vi "SPARC4_GEI.vi"() -> ()   [LabVIEW 2018]
uses:
  SPARC4_GUI/SPARC4_GEI.lvclass
  SPARC4_GUI/SPARC4_GEI.lvclass/SPARC4_GEI.ctl
  Interface/Interface.lvclass/Interface.ctl
  Channel GUI/Channel GEI.lvclass/Channel GEI.ctl
  State Machine/State Machine.lvclass/State Machine.ctl
  Channel GUI/Channel GEI.lvclass
  State Machine/State Machine.lvclass
  RxTx/RxTx.lvclass
  Interface/Interface.lvclass
panel:
  out "Error Message":string
  in  "Tab Control 2":enum32{"Front Panel", "Setup Panel"}(tab)
  in  "Number of channels":u16=1 min=1
  in  "FOCUS":bool caption="TEST"
  in  "TEST":bool
  in  "ZERO":bool caption="BIAS"
  in  "FLAT":bool
  in  "OBJECT":bool caption="SCIENCE"
  in  "DARK":bool caption="TEST"
  in  "Suffix:":string
  in  "Comment:":string="Go SPARC4!"
  in  "Filter":u16(ring) items=["Clear", "U", "B", "V", "R", "I"]
  out "Exposições realizadas":u16(slide)=1 max=2 scale=0.0..1.0
  out "Exposing":bool
  in  "Dummy":bool
  out "Camera On/Off":bool
  in  "Abort Acquisition":bool
  in  "Stop Acquisition":bool
  in  "Cubes":u32=1 min=1
  in  "Frames":u16=1 min=1
  in  "Send Message":bool
  out "Response:":string
  in  "Command:":string
  out "Last image":string="CH1"
  out "CCD Status":string
  out "Exp Time":sgl
  out "Temperature":i16
  out "Serial Number":u16
  out "Temperature Status":string
  in  "Exposure Time":sgl=1.0 min=1e-05
  in  "Acquire":bool
  in  "Stop Application":bool
  in  "TCS Simulated/Real":bool
  in  "EM Mode":u8(ring)=1 items=["Electron Multiplying", "Conventional"]
  in  "EM Gain":u16=2
  in  "Temperature 2":i16=20 min=-80 max=20
  in  "Cooler ON/OFF":u16(ring) items=["Cooler OFF", "Cooler ON"]
  in  "Readout Rate":u8(ring) items=["1 MHz", "0.1 MHz"]
  in  "Exposure Time 2":sgl=1.0 min=1e-05
  in  "Pre-amp gain":u8(ring) items=["Gain 1", "Gain 2"]
  in  "Frames 2":u16=1 min=1
  in  "Frame Tansfer":bool=TRUE
  in  "Trigger Mode":u16(ring) items=["Internal", "External", "N/A", "N/A", "N/A", "N/A", "External Start", "External Exposure (Bulb)", "N/A", "External FVB EM", "Software", "N/A", "External Charge Shifting"]
  in  "Vertical Shift Speed":u16=3
  in  "Read Mode":u16(ring)=4 items=["Full Vertical Binning", "Multi-Track", "Random-Track", "Single-Track", "Image"]
  in  "Vertical Clock Voltagem":u16
  in  "AD Channel":u16
  in  "Acquisition Mode":u16(ring)=3 items=["Reserved", "Single Scan", "Accumulate", "Kinetic", "Fast Kinetic", "Run till abort", "Reserved", "Reserved", "Reserved", "Time Delayed Integration"]
  in  "Shutter TTL":u16(ring) items=["TTL Low", "TTL High"]
  in  "Shutter Time":u16=50
  in  "Shutter Mode":u8(ring)=2 items=["Fully Auto", "OPEN", "CLOSED"]
  in  "Sub Image":T1(radio)=enum."1024 x 1024"
  in  "Final Line":u16=1024
  in  "Final Column":u16=1024
  in  "Initial Cloumn":u16=1
  in  "Initial Line":u16=1
  in  "Binning":u16=1
  # "SPARC4  ACS\nGraphical Engineering Interface (GEI)"
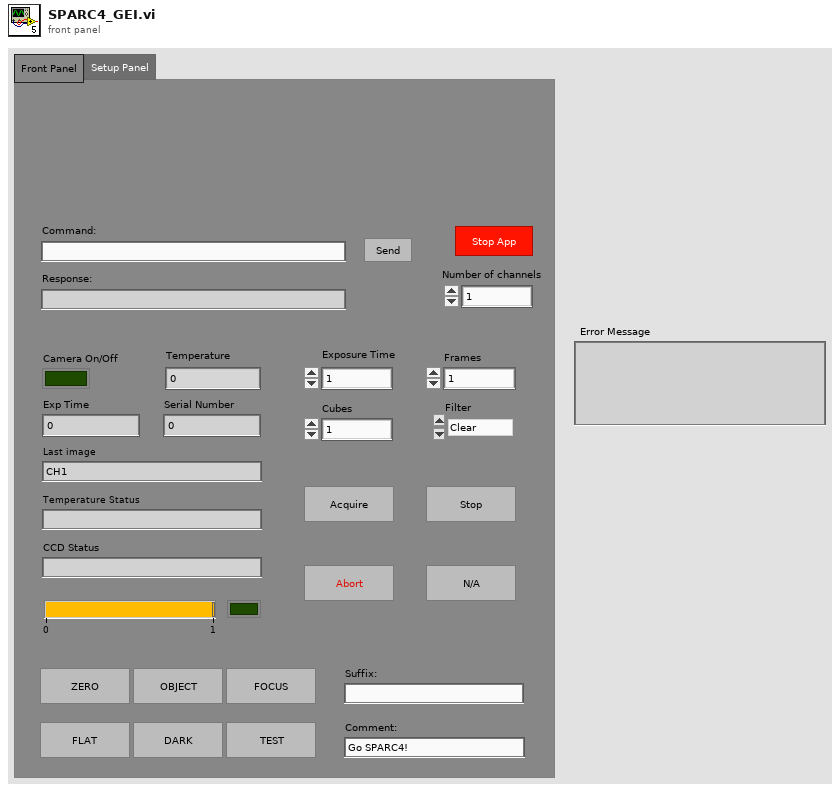
[diagram p1: front panel]
types:
  T1 = enum32{"256 x 256", "512 x 512", "1024 x 1024", "Custom"}
  T2 = enum8{"Enabled", "Disabled", "Disabled and Grayed Out"}
  T3 = cluster{"CUBE_EXPOSURE_TIME":sgl, "CUBES_DONE":u16, "LAST_IMAGE_NAME":string, "DISK_SPACE":u16, "FRAMES_DONE":u16, "CCD_STATUS":string, "CURRENT_TEMPERATURE":i16, "TEMPERATURE_STATUS":string, "FRAME_EXPOSURE_TIME":dbl, "CCD_POWER_STATUS":bool, "SERIAL_NUMBER":u16, "ACQUIRING":bool}
  T4 = cluster{"PREAMP":u16, "READOUT_RATE":u16, "EM_GAIN":u16, "VBIN":u16, "INITIAL_LINE":u16, "INITIAL_COLUMN":u16, "FINAL_LINE":u16, "FINAL_COLUMN":u16, "TRIGGER_MODE":u16, "HBIN":u16, "SHUTTER_TTL":u16, "SHUTTER_MODE":u16, "SHUTTER_OPENING_TIME":u16, "SHUTTER_CLOSING_TIME":u16, "VERTICAL_SHIFT_SPEED":u16, "READ_MODE":u16, "FRAME_TRANSFER":bool, "VERTICAL_CLOCK_VOLTAGE":u16, "ACQUISITION_MODE":u16, "AD_CHANNEL":u16, "EM_MODE":u16}
  T5 = cluster{"COOLER_POWER_STATUS":u16, "TEMP":i32, "EXPTIME":dbl, "#FRAMES":u32, "#CUBES":u32}
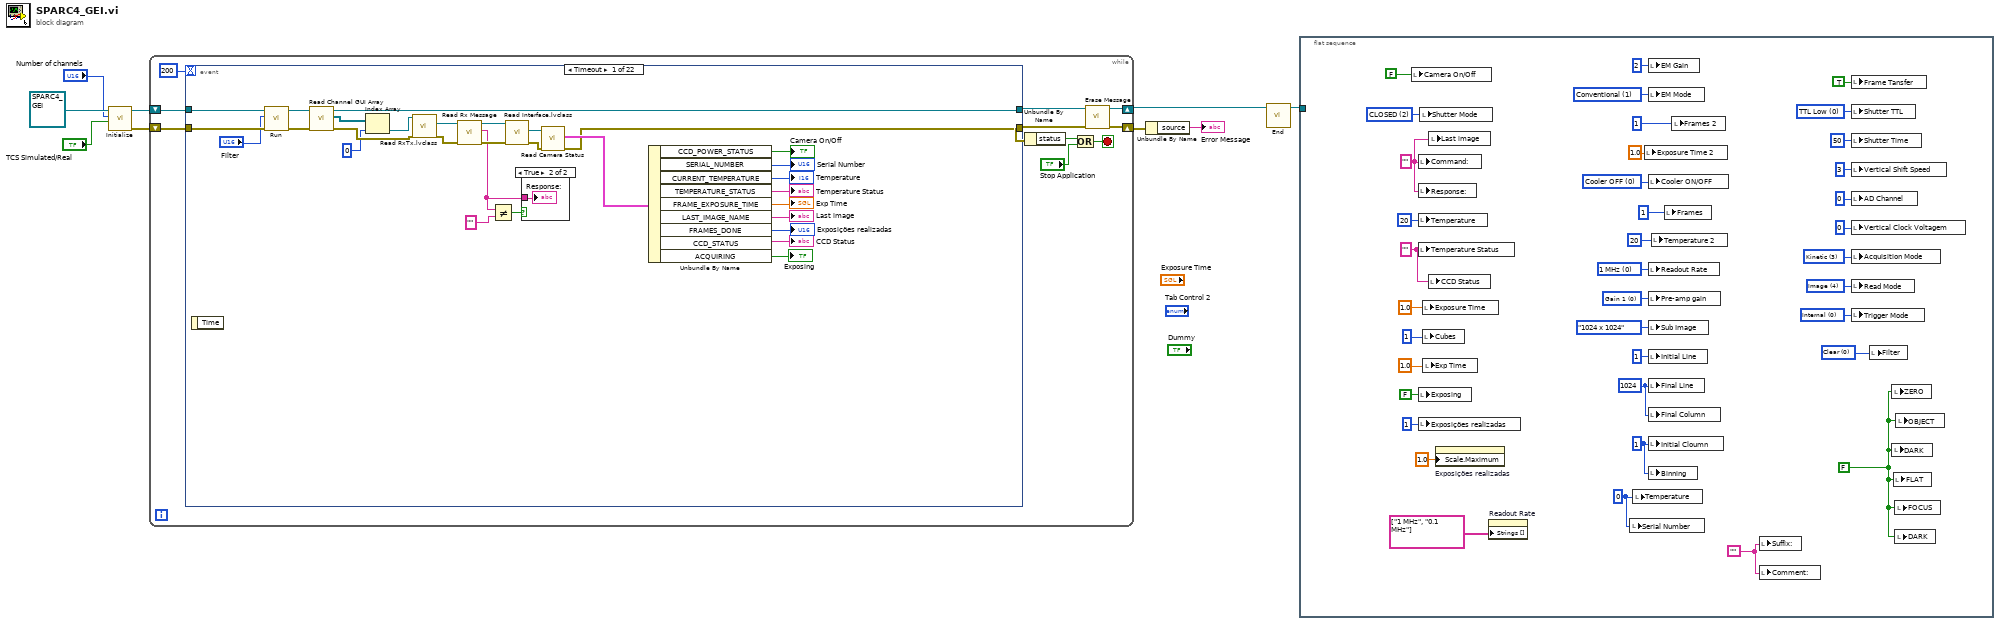
[diagram p0: block diagram]
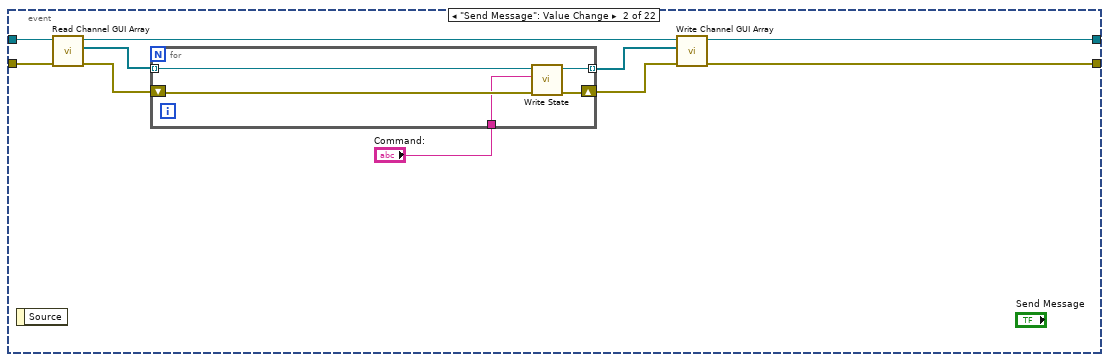
[diagram p3: hidden frame]
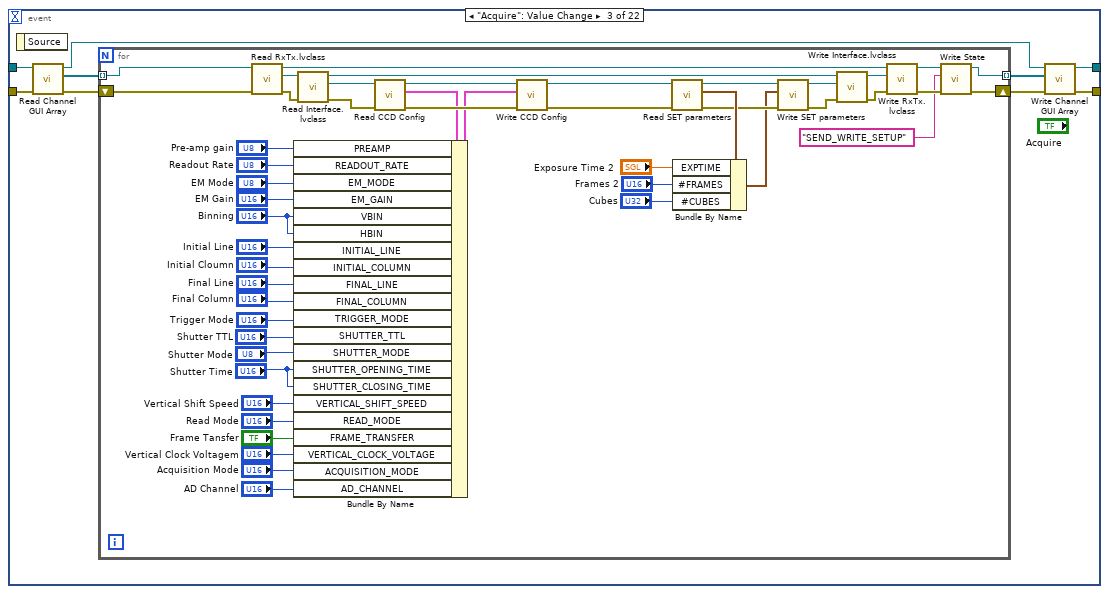
[diagram p4: hidden frame]
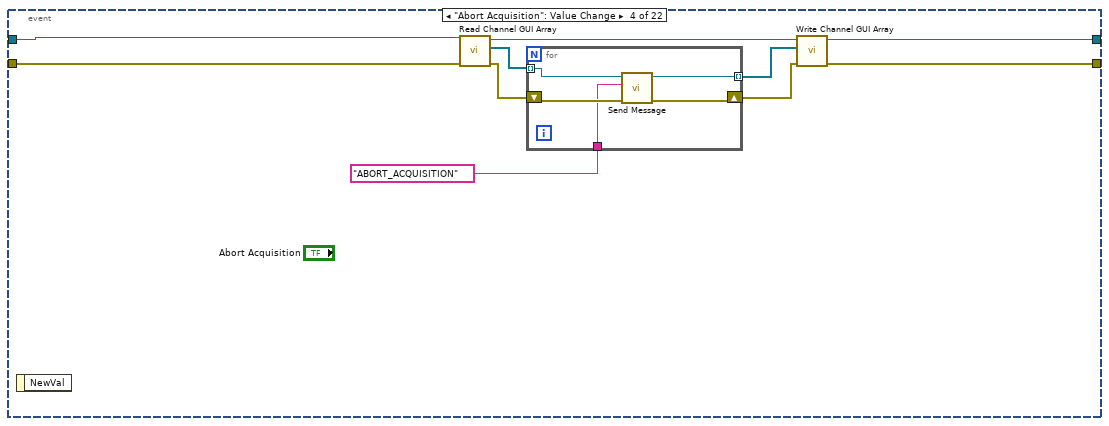
[diagram p5: hidden frame]
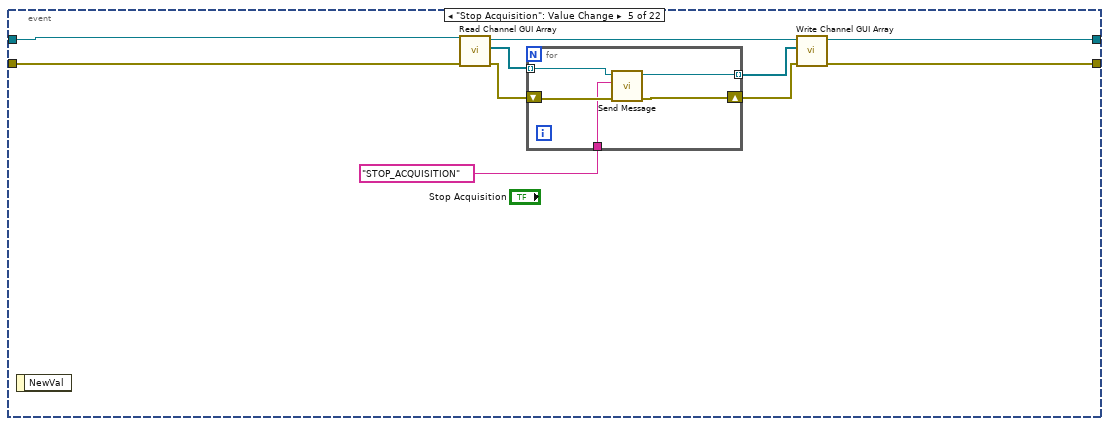
[diagram p6: hidden frame]
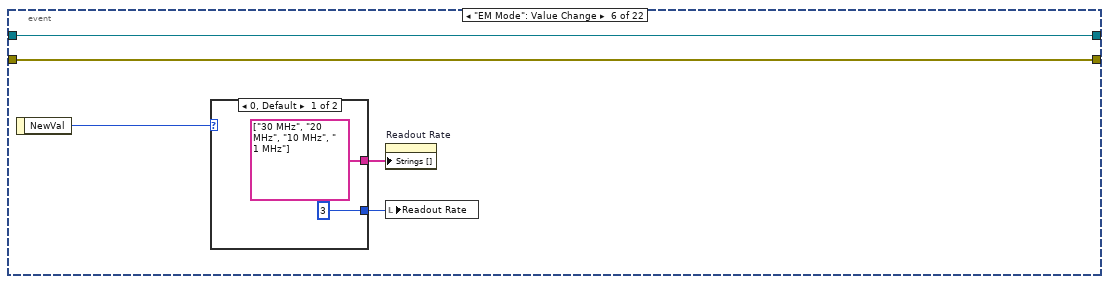
[diagram p7: hidden frame]
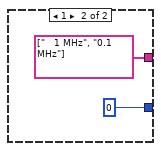
[diagram p8: hidden frame]
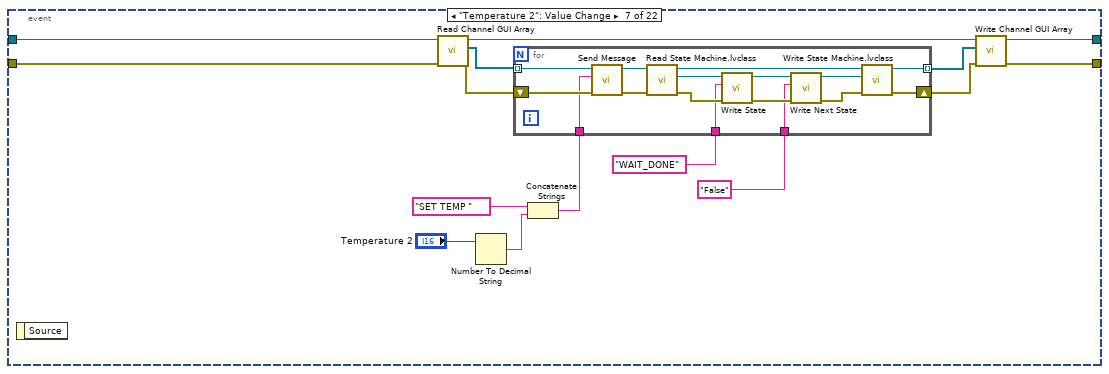
[diagram p9: hidden frame]
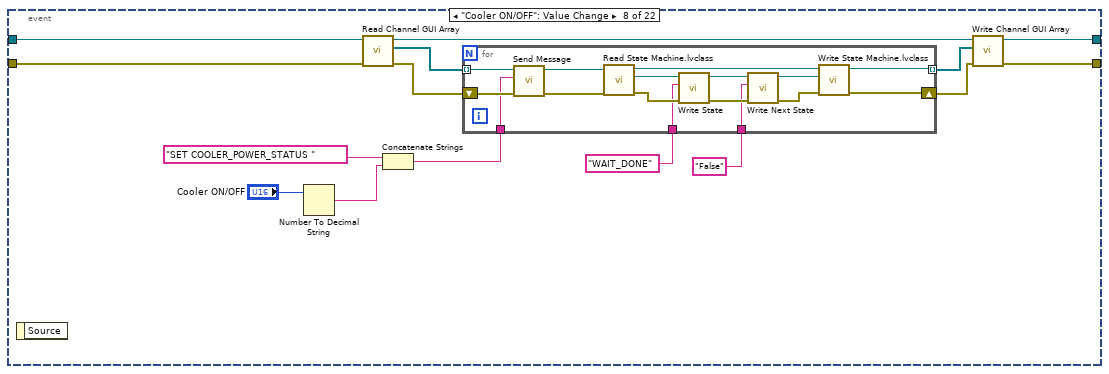
[diagram p10: hidden frame]
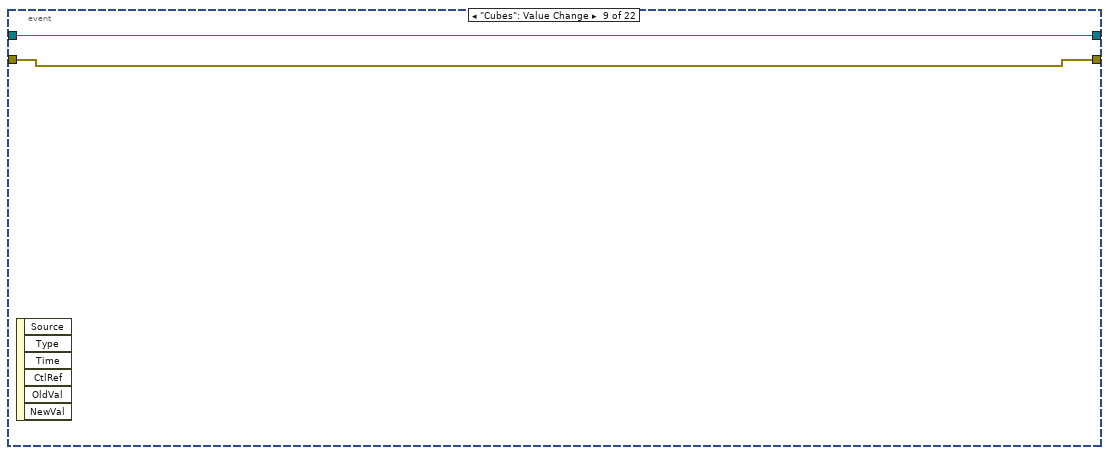
[diagram p11: hidden frame]
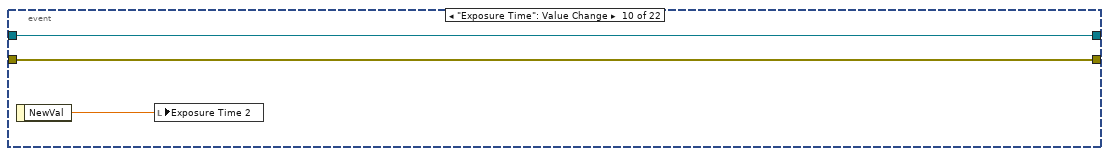
[diagram p12: hidden frame]
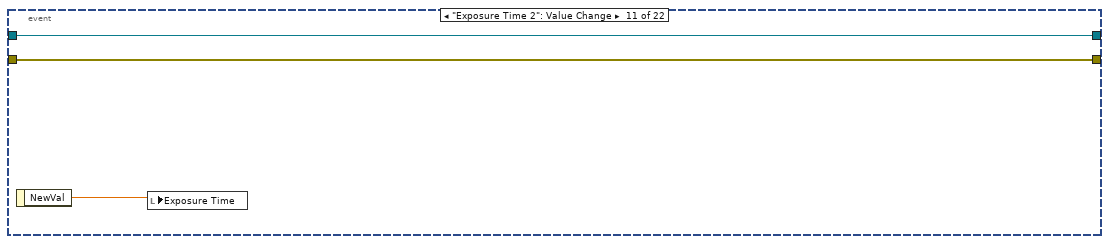
[diagram p13: hidden frame]
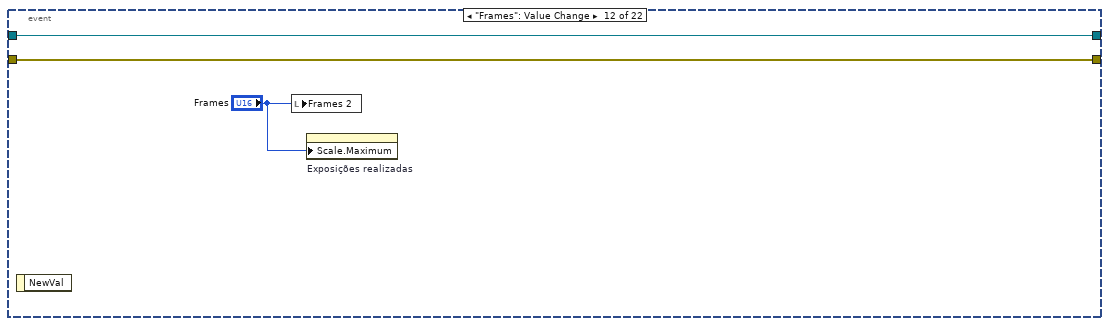
[diagram p14: hidden frame]
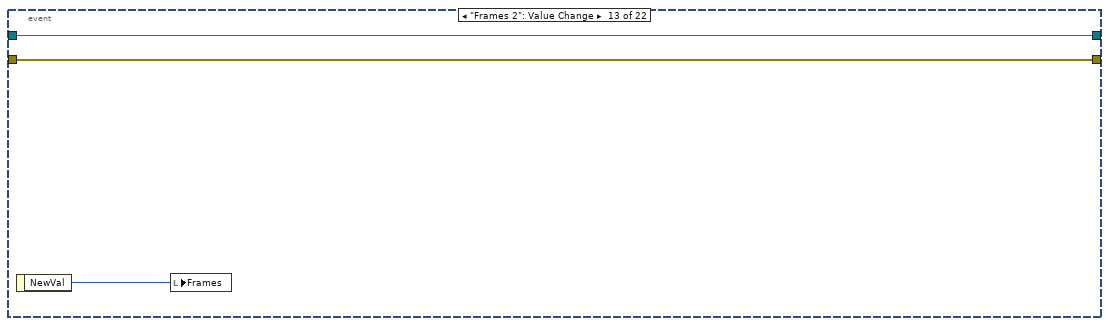
[diagram p15: hidden frame]
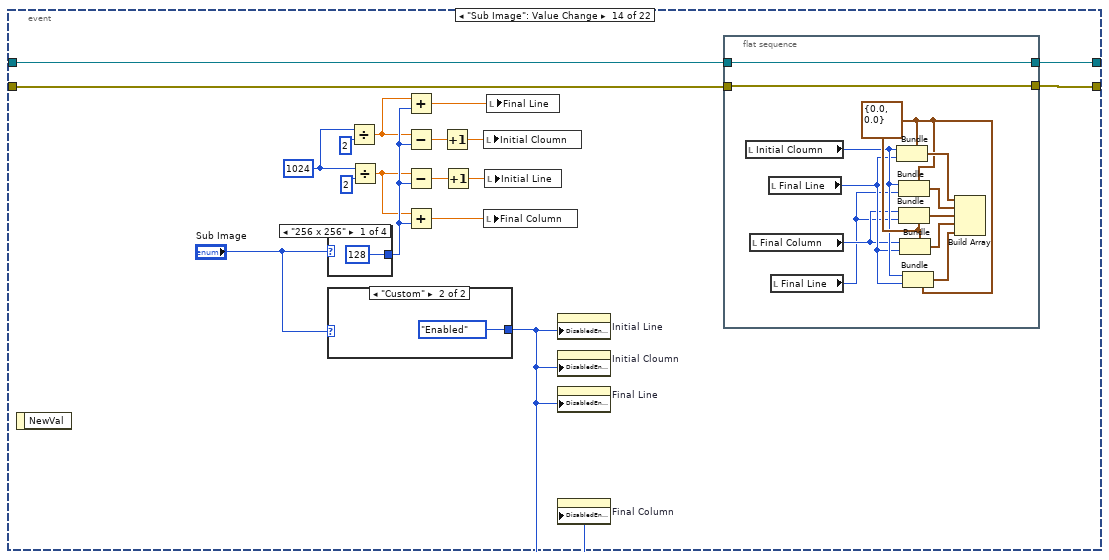
[diagram p16: hidden frame]
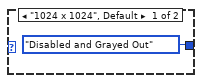
[diagram p17: hidden frame]
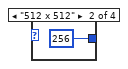
[diagram p18: hidden frame]
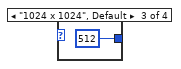
[diagram p19: hidden frame]
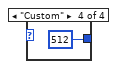
[diagram p20: hidden frame]
diagram:
  n1 = call "Initialize.vi"("TCS Simulated/Real"="TCS Simulated/Real", "channels quantity"="Number of channels", "SPARC4_GUI in"=refnum<class "SPARC4_GEI.lvclass"> refnum ("SPARC4_GUI.lvclass")) -> ("error out"=w9:errorcluster, "SPARC4_GUI out"=w8:refnum<class "SPARC4_GEI.lvclass">)  [unwired: 7 in]
  n2 = while {
    shift-right: [w13] -> w4
    shift-left: w9 -> [w14]
    shift-right: [w12] -> w5
    shift-left: w8 -> [w15]
    stop <- w18 stop-if-true
    n3 = event shown="[0] Timeout" {
      selector: _ -> [_ _ _ _ _ _ _ _ _ _ _ _ _ _ _ _ _ _ _ _ _ _]
      dyn-events: _ -> [_ _ _ _ _ _ _ _ _ _ _ _ _ _ _ _ _ _ _ _ _ _]
      timeout: 200 -> [_ _ _ _ _ _ _ _ _ _ _ _ _ _ _ _ _ _ _ _ _ _]
      tunnel: w14 -> [w46 w59 w73 w128 w143 w157 w168 w200 w225 w228 w231 w234 w237 w255 w280 w310 w349 w393 w437 w481 w525 w567]
      tunnel: [w27 w51 w66 w126 w141 w157 w173 w198 w225 w228 w231 w234 w237 w253 w278 w308 w347 w391 w435 w479 w523 w565] -> w10
      tunnel: w15 -> [w47 w60 w74 w129 w144 w158 w167 w201 w226 w229 w230 w235 w238 w256 w281 w311 w350 w394 w438 w482 w526 w568]
      tunnel: [w39 w52 w67 w127 w142 w158 w174 w199 w226 w229 w230 w235 w238 w254 w279 w309 w348 w392 w436 w480 w524 w566] -> w11
      event Timeout {
        n4 = event-data() -> ()  [unwired: 1 in, 1 out]
        n5 = call "Run.vi"("error in (no error)"=w46, "Filter"="Filter", "SPARC4_GUI in"=w47) -> ("error out"=w49:errorcluster, "SPARC4_GUI out"=w48:refnum<class "SPARC4_GEI.lvclass">)  [unwired: 7 in]
        n6 = call "Read Channel GUI Array.vi"("error in (no error)"=w49, "SPARC4_GUI in"=w48) -> ("error out"=w41:errorcluster, "Channel GUI Array"=w43:refnum<class "Channel GEI.lvclass">[], "SPARC4_GUI out"=w39:refnum<class "SPARC4_GEI.lvclass">)  [unwired: 7 in]
        n7 = Index Array(array=w43, index=0) -> (element=w42:refnum<class "Channel GEI.lvclass">)
        n8 = call "Read RxTx.lvclass.vi"("error in (no error)"=w41, "Channel GUI in"=w42) -> ("error out"=w40:errorcluster, "RxTx.lvclass"=w38:refnum<class "RxTx.lvclass">)  [unwired: 7 in, 1 out]
        n9 = call "Read Rx Message.vi"("error in (no error)"=w40, "RxTx in"=w38) -> ("error out"=w44:errorcluster, "Rx Message"=w24:string, "RxTx out"=w45:refnum<class "RxTx.lvclass">)  [unwired: 7 in]
        n10 = Not Equal?(x=w24, y="") -> (x != y?=w25:bool)
        n11 = call "Read Interface.lvclass.vi"("error in (no error)"=w44, "RxTx in"=w45) -> ("error out"=w29:errorcluster, "Interface.lvclass"=w30:refnum<class "Interface.lvclass">)  [unwired: 7 in, 1 out]
        n12 = case shown="True" w25 {
          tunnel: w24 -> [_ w50]
          frame False {
          }
          frame True {
            "Response:" <- w50
          }
        }
        n13 = call "Read Camera Status.vi"("error in (no error)"=w29, "Interface in"=w30) -> ("error out"=w27:errorcluster, "Camera Status"=w28:T3)  [unwired: 7 in, 1 out]
        n14 = Unbundle By Name(w28) -> ("CCD_POWER_STATUS"=→"Camera On/Off":bool, "SERIAL_NUMBER"=→"Serial Number":u16, "CURRENT_TEMPERATURE"=→"Temperature":i16, "TEMPERATURE_STATUS"=→"Temperature Status":string, "FRAME_EXPOSURE_TIME"=→"Exp Time":dbl, "LAST_IMAGE_NAME"=→"Last image":string, "FRAMES_DONE"=→"Exposições realizadas":u16, "CCD_STATUS"=→"CCD Status":string, "ACQUIRING"=→"Exposing":bool)
      }
      event "Send Message": Value Change {
        n15 = event-data() -> ()  [unwired: 1 in, 1 out]
        n16 = call "Read Channel GUI Array.vi"("error in (no error)"=w59, "SPARC4_GUI in"=w60) -> ("error out"=w56:errorcluster, "Channel GUI Array"=w58:refnum<class "Channel GEI.lvclass">[], "SPARC4_GUI out"=w55:refnum<class "SPARC4_GEI.lvclass">)  [unwired: 7 in]
        n17 = for {
          tunnel: w58 -> [w65] mode=indexing
          shift-right: [w63] -> w57
          shift-left: w56 -> [w64]
          tunnel: [w62] -> w54 mode=indexing
          tunnel: "Command:" -> [w61]
          n18 = call "Write State.vi"("error in (no error)"=w64, "State"=w61, "Channel GEI in"=w65) -> ("error out"=w63:errorcluster, "Channel GEI out"=w62:refnum<class "Channel GEI.lvclass">)  [unwired: 7 in]
        }
        n19 = call "Write Channel GUI Array.vi"("error in (no error)"=w57, "Channel GUI Array"=w54, "SPARC4_GUI in"=w55) -> ("error out"=w51:errorcluster, "SPARC4_GUI out"=w52:refnum<class "SPARC4_GEI.lvclass">)  [unwired: 7 in]
      }
      event "Acquire": Value Change {
        n20 = event-data() -> ()  [unwired: 1 in, 1 out]
        n21 = call "Read Channel GUI Array.vi"("error in (no error)"=w73, "SPARC4_GUI in"=w74) -> ("error out"=w71:errorcluster, "Channel GUI Array"=w72:refnum<class "Channel GEI.lvclass">[], "SPARC4_GUI out"=w69:refnum<class "SPARC4_GEI.lvclass">)  [unwired: 7 in]
        n22 = for {
          tunnel: w72 -> [w119] mode=indexing
          shift-right: [w113] -> w70
          shift-left: w71 -> [w118]
          tunnel: [w114] -> w68 mode=indexing
          n23 = call "Read RxTx.lvclass.vi"("error in (no error)"=w118, "Channel GUI in"=w119) -> ("error out"=w122:errorcluster, "RxTx.lvclass"=w117:refnum<class "RxTx.lvclass">, "Channel GUI out"=w120:refnum<class "Channel GEI.lvclass">)  [unwired: 7 in]
          n24 = call "Read Interface.lvclass.vi"("error in (no error)"=w122, "RxTx in"=w117) -> ("error out"=w107:errorcluster, "Interface.lvclass"=w110:refnum<class "Interface.lvclass">, "RxTx out"=w123:refnum<class "RxTx.lvclass">)  [unwired: 7 in]
          n25 = call "Read CCD Config.vi"("error in (no error)"=w107, "Interface in"=w110) -> ("error out"=w108:errorcluster, "Previous CCD Config"=w88:T4, "Interface out"=w109:refnum<class "Interface.lvclass">)  [unwired: 7 in]
          n26 = Bundle By Name(cluster=w88, "PREAMP"="Pre-amp gain", "READOUT_RATE"="Readout Rate", "EM_MODE"="EM Mode", "EM_GAIN"="EM Gain", "VBIN"="Binning", "HBIN"="Binning", "INITIAL_LINE"="Initial Line", "INITIAL_COLUMN"="Initial Cloumn", "FINAL_LINE"="Final Line", "FINAL_COLUMN"="Final Column", "TRIGGER_MODE"="Trigger Mode", "SHUTTER_TTL"="Shutter TTL", "SHUTTER_MODE"="Shutter Mode", "SHUTTER_OPENING_TIME"="Shutter Time", "SHUTTER_CLOSING_TIME"="Shutter Time", "VERTICAL_SHIFT_SPEED"="Vertical Shift Speed", "READ_MODE"="Read Mode", "FRAME_TRANSFER"="Frame Tansfer", "VERTICAL_CLOCK_VOLTAGE"="Vertical Clock Voltagem", "ACQUISITION_MODE"="Acquisition Mode", "AD_CHANNEL"="AD Channel") -> (w87:T4)
          n27 = call "Write CCD Config.vi"("error in (no error)"=w108, "CCD Config"=w87, "Interface in"=w109) -> ("error out"=w85:errorcluster, "Interface out"=w86:refnum<class "Interface.lvclass">)  [unwired: 7 in]
          n28 = call "Read SET parameters.vi"("error in (no error)"=w85, "Interface in"=w86) -> ("error out"=w82:errorcluster, "SET parameters"=w84:T5, "Interface out"=w83:refnum<class "Interface.lvclass">)  [unwired: 7 in]
          n29 = Bundle By Name(cluster=w84, "EXPTIME"="Exposure Time 2", "#FRAMES"="Frames 2", "#CUBES"="Cubes") -> (w79:T5)
          n30 = call "Write SET parameters.vi"("error in (no error)"=w82, "SET parameters"=w79, "Interface in"=w83) -> ("error out"=w81:errorcluster, "Interface out"=w80:refnum<class "Interface.lvclass">)  [unwired: 7 in]
          n31 = call "Write Interface.lvclass.vi"("error in (no error)"=w81, "Interface.lvclass"=w80, "RxTx in"=w123) -> ("error out"=w121:errorcluster, "RxTx out"=w116:refnum<class "RxTx.lvclass">)  [unwired: 7 in]
          n32 = call "Write RxTx.lvclass.vi"("error in (no error)"=w121, "RxTx.lvclass"=w116, "Channel GUI in"=w120) -> ("error out"=w112:errorcluster, "Channel GUI out"=w115:refnum<class "Channel GEI.lvclass">)  [unwired: 7 in]
          n33 = call "Write State.vi"("error in (no error)"=w112, "State"="SEND_WRITE_SETUP", "Channel GEI in"=w115) -> ("error out"=w113:errorcluster, "Channel GEI out"=w114:refnum<class "Channel GEI.lvclass">)  [unwired: 7 in]
        }
        n34 = call "Write Channel GUI Array.vi"("error in (no error)"=w70, "Channel GUI Array"=w68, "SPARC4_GUI in"=w69) -> ("error out"=w66:errorcluster, "SPARC4_GUI out"=w67:refnum<class "SPARC4_GEI.lvclass">)  [unwired: 7 in]
      }
      event "Abort Acquisition": Value Change {
        n35 = event-data() -> ()  [unwired: 1 in, 1 out]
        n36 = call "Read Channel GUI Array.vi"("error in (no error)"=w128, "SPARC4_GUI in"=w129) -> ("error out"=w130:errorcluster, "Channel GUI Array"=w132:refnum<class "Channel GEI.lvclass">[], "SPARC4_GUI out"=w133:refnum<class "SPARC4_GEI.lvclass">)  [unwired: 7 in]
        n37 = for {
          tunnel: w132 -> [w138] mode=indexing
          shift-right: [w136] -> w131
          shift-left: w130 -> [w135]
          tunnel: "ABORT_ACQUISITION" ("Message") -> [w134]
          tunnel: [w137] -> w124 mode=indexing
          n38 = call "Send Message.vi"("error in (no error)"=w135, "Message"=w134, "Channel GUI in"=w138) -> ("error out"=w136:errorcluster, "Channel GUI out"=w137:refnum<class "Channel GEI.lvclass">)  [unwired: 7 in]
        }
        n39 = call "Write Channel GUI Array.vi"("error in (no error)"=w131, "Channel GUI Array"=w124, "SPARC4_GUI in"=w133) -> ("error out"=w126:errorcluster, "SPARC4_GUI out"=w127:refnum<class "SPARC4_GEI.lvclass">)  [unwired: 7 in]
      }
      event "Stop Acquisition": Value Change {
        n40 = event-data() -> ()  [unwired: 1 in, 1 out]
        n41 = call "Read Channel GUI Array.vi"("error in (no error)"=w143, "SPARC4_GUI in"=w144) -> ("error out"=w145:errorcluster, "Channel GUI Array"=w147:refnum<class "Channel GEI.lvclass">[], "SPARC4_GUI out"=w148:refnum<class "SPARC4_GEI.lvclass">)  [unwired: 7 in]
        n42 = for {
          tunnel: w147 -> [w151] mode=indexing
          shift-right: [w153] -> w146
          shift-left: w145 -> [w150]
          tunnel: "STOP_ACQUISITION" ("Message") -> [w149]
          tunnel: [w152] -> w139 mode=indexing
          n43 = call "Send Message.vi"("error in (no error)"=w150, "Message"=w149, "Channel GUI in"=w151) -> ("error out"=w153:errorcluster, "Channel GUI out"=w152:refnum<class "Channel GEI.lvclass">)  [unwired: 7 in]
        }
        n44 = call "Write Channel GUI Array.vi"("error in (no error)"=w146, "Channel GUI Array"=w139, "SPARC4_GUI in"=w148) -> ("error out"=w141:errorcluster, "SPARC4_GUI out"=w142:refnum<class "SPARC4_GEI.lvclass">)  [unwired: 7 in]
      }
      event "EM Mode": Value Change {
        n45 = event-data() -> ("NewVal"=w155:u8)  [unwired: 1 in]
        n46 = case shown="0, Default" w155 {
          tunnel: [string[] ["30 MHz", "20 MHz", "10 MHz", "  1 MHz"] string[] ["   1 MHz", "0.1 MHz"]] -> w156
          tunnel: [3 0] -> w154
          frame 0, Default {
          }
          frame 1 {
          }
        }
        n47 = property on="Readout Rate" class="Ring (strict)"("Strings []"=w156) -> ()  [unwired: 2 in, 2 out]
        n48 = local write "Readout Rate"(w154) -> ()
      }
      event "Temperature 2": Value Change {
        n49 = event-data() -> ()  [unwired: 1 in, 1 out]
        n50 = call "Read Channel GUI Array.vi"("error in (no error)"=w168, "SPARC4_GUI in"=w167) -> ("error out"=w169:errorcluster, "Channel GUI Array"=w170:refnum<class "Channel GEI.lvclass">[], "SPARC4_GUI out"=w171:refnum<class "SPARC4_GEI.lvclass">)  [unwired: 7 in]
        n51 = Number To Decimal String(number="Temperature 2") -> (decimal integer string=w176:string)  [unwired: 1 in]
        n52 = Concatenate Strings("SET TEMP " ("Message"), w176) -> (w166:string)
        n53 = for {
          tunnel: w170 -> [w192] mode=indexing
          shift-right: [w188] -> w172
          shift-left: w169 -> [w193]
          tunnel: w166 -> [w191]
          tunnel: [w187] -> w165 mode=indexing
          tunnel: "WAIT_DONE" ("Message") -> [w179]
          tunnel: "False" ("Message") -> [w178]
          n54 = call "Send Message.vi"("error in (no error)"=w193, "Message"=w191, "Channel GUI in"=w192) -> ("error out"=w189:errorcluster, "Channel GUI out"=w190:refnum<class "Channel GEI.lvclass">)  [unwired: 7 in]
          n55 = call "Read State Machine.lvclass.vi"("error in (no error)"=w189, "Channel GUI in"=w190) -> ("error out"=w181:errorcluster, "State Machine.lvclass"=w186:refnum<class "State Machine.lvclass">, "Channel GUI out"=w180:refnum<class "Channel GEI.lvclass">)  [unwired: 7 in]
          n56 = call-dynamic "Write State.vi"("error in (no error)"=w181, "State"=w179, "State Machine in"=w186) -> ("error out"=w182:errorcluster, "State Machine out"=w185:refnum<class "State Machine.lvclass">)  [unwired: 7 in]
          n57 = call "Write Next State.vi"("error in (no error)"=w182, "Next State"=w178, "State Machine in"=w185) -> ("error out"=w183:errorcluster, "State Machine out"=w184:refnum<class "State Machine.lvclass">)  [unwired: 7 in]
          n58 = call "Write State Machine.lvclass.vi"("error in (no error)"=w183, "State Machine.lvclass"=w184, "Channel GUI in"=w180) -> ("error out"=w188:errorcluster, "Channel GUI out"=w187:refnum<class "Channel GEI.lvclass">)  [unwired: 7 in]
        }
        n59 = call "Write Channel GUI Array.vi"("error in (no error)"=w172, "Channel GUI Array"=w165, "SPARC4_GUI in"=w171) -> ("error out"=w173:errorcluster, "SPARC4_GUI out"=w174:refnum<class "SPARC4_GEI.lvclass">)  [unwired: 7 in]
      }
      event "Cooler ON/OFF": Value Change {
        n60 = event-data() -> ()  [unwired: 1 in, 1 out]
        n61 = Number To Decimal String(number="Cooler ON/OFF") -> (decimal integer string=w206:string)  [unwired: 1 in]
        n62 = call "Read Channel GUI Array.vi"("error in (no error)"=w200, "SPARC4_GUI in"=w201) -> ("error out"=w202:errorcluster, "Channel GUI Array"=w203:refnum<class "Channel GEI.lvclass">[], "SPARC4_GUI out"=w204:refnum<class "SPARC4_GEI.lvclass">)  [unwired: 7 in]
        n63 = Concatenate Strings("SET COOLER_POWER_STATUS ", w206) -> (w197:string)
        n64 = for {
          tunnel: w203 -> [w224] mode=indexing
          shift-right: [w211] -> w205
          shift-left: w202 -> [w223]
          tunnel: w197 -> [w222]
          tunnel: [w212] -> w196 mode=indexing
          tunnel: "WAIT_DONE" ("Message") -> [w210]
          tunnel: "False" ("Message") -> [w209]
          n65 = call "Send Message.vi"("error in (no error)"=w223, "Message"=w222, "Channel GUI in"=w224) -> ("error out"=w213:errorcluster, "Channel GUI out"=w214:refnum<class "Channel GEI.lvclass">)  [unwired: 7 in]
          n66 = call "Read State Machine.lvclass.vi"("error in (no error)"=w213, "Channel GUI in"=w214) -> ("error out"=w220:errorcluster, "State Machine.lvclass"=w215:refnum<class "State Machine.lvclass">, "Channel GUI out"=w221:refnum<class "Channel GEI.lvclass">)  [unwired: 7 in]
          n67 = call-dynamic "Write State.vi"("error in (no error)"=w220, "State"=w210, "State Machine in"=w215) -> ("error out"=w219:errorcluster, "State Machine out"=w216:refnum<class "State Machine.lvclass">)  [unwired: 7 in]
          n68 = call "Write Next State.vi"("error in (no error)"=w219, "Next State"=w209, "State Machine in"=w216) -> ("error out"=w218:errorcluster, "State Machine out"=w217:refnum<class "State Machine.lvclass">)  [unwired: 7 in]
          n69 = call "Write State Machine.lvclass.vi"("error in (no error)"=w218, "State Machine.lvclass"=w217, "Channel GUI in"=w221) -> ("error out"=w211:errorcluster, "Channel GUI out"=w212:refnum<class "Channel GEI.lvclass">)  [unwired: 7 in]
        }
        n70 = call "Write Channel GUI Array.vi"("error in (no error)"=w205, "Channel GUI Array"=w196, "SPARC4_GUI in"=w204) -> ("error out"=w198:errorcluster, "SPARC4_GUI out"=w199:refnum<class "SPARC4_GEI.lvclass">)  [unwired: 7 in]
      }
      event "Cubes": Value Change {
        n71 = event-data() -> ()  [unwired: 1 in, 6 out]
      }
      event "Exposure Time": Value Change {
        n72 = event-data() -> ("NewVal"=w227:sgl)  [unwired: 1 in]
        n73 = local write "Exposure Time 2"(w227) -> ()
      }
      event "Exposure Time 2": Value Change {
        n74 = event-data() -> ("NewVal"=w232:sgl)  [unwired: 1 in]
        n75 = local write "Exposure Time"(w232) -> ()
      }
      event "Frames": Value Change {
        n76 = event-data() -> ()  [unwired: 1 in, 1 out]
        n77 = local write "Frames 2"("Frames") -> ()
        n78 = property on="Exposições realizadas" class="Slide (strict)"("Scale.Maximum"="Frames") -> ()  [unwired: 2 in, 2 out]
      }
      event "Frames 2": Value Change {
        n79 = event-data() -> ("NewVal"=w236:u16)  [unwired: 1 in]
        n80 = local write "Frames"(w236) -> ()
      }
      event "Sub Image": Value Change {
        w243 = 1024
        n81 = event-data() -> ()  [unwired: 1 in, 1 out]
        n82 = case shown="\"256 x 256\"" "Sub Image" {
          tunnel: [128 256 512 512] -> w247
          frame "256 x 256" {
          }
          frame "512 x 512" {
          }
          frame "1024 x 1024", Default {
          }
          frame "Custom" {
          }
        }
        n83 = case shown="\"Custom\"" "Sub Image" {
          tunnel: [T2."Disabled and Grayed Out" ("Disabled") T2."Enabled" ("Disabled")] -> w250
          frame "1024 x 1024", Default {
          }
          frame "Custom" {
          }
        }
        n84 = Divide(x=w243, y=2) -> (x/y=w246:dbl)
        n85 = Divide(x=w243, y=2) -> (x/y=w245:dbl)
        n86 = Add(x=w246, y=w247) -> (x+y=w239:dbl)
        n87 = Subtract(x=w246, y=w247) -> (x-y=w248:dbl)
        n88 = Subtract(x=w245, y=w247) -> (x-y=w249:dbl)
        n89 = Add(x=w245, y=w247) -> (x+y=w252:dbl)
        n90 = Increment(x=w248) -> (x+1=w251:dbl)
        n91 = Increment(x=w249) -> (x+1=w240:dbl)
        n92 = local write "Initial Cloumn"(w251) -> ()
        n93 = local write "Final Column"(w252) -> ()
        n94 = local write "Initial Line"(w240) -> ()
        n95 = local write "Final Line"(w239) -> ()
        n96 = property on="Initial Line" class="DigNum (strict)"("DisabledEnum"=w250) -> ()  [unwired: 2 in, 2 out]
        n97 = property on="Initial Cloumn" class="DigNum (strict)"("DisabledEnum"=w250) -> ()  [unwired: 2 in, 2 out]
        n98 = property on="Final Line" class="DigNum (strict)"("DisabledEnum"=w250) -> ()  [unwired: 2 in, 2 out]
        n99 = property on="Final Column" class="DigNum (strict)"("DisabledEnum"=w250) -> ()  [unwired: 2 in, 2 out]
        n100 = flat-sequence {
          tunnel: w255 -> [w273]
          tunnel: w256 -> [w274]
          tunnel: [w274] -> w254
          tunnel: [w273] -> w253
          frame #0 {
            w267 = cluster{dbl, dbl} {0.0, 0.0}
            n101 = local read "Initial Cloumn"() -> (w266:u16)
            n102 = local read "Final Column"() -> (w264:u16)
            n103 = local read "Final Line"() -> (w265:u16)
            n104 = local read "Final Line"() -> (w263:u16)
            n105 = Bundle(cluster=w267, w266, w265) -> (w272:cluster{dbl, dbl})
            n106 = Bundle(cluster=w267, w266, w263) -> (w271:cluster{dbl, dbl})
            n107 = Bundle(cluster=w267, w264, w263) -> (w270:cluster{dbl, dbl})
            n108 = Bundle(cluster=w267, w264, w265) -> (w269:cluster{dbl, dbl})
            n109 = Bundle(cluster=w267, w266, w265) -> (w268:cluster{dbl, dbl})
            n110 = Build Array(w272, w271, w270, w269, w268) -> ()  [unwired: 1 out]
          }
        }
      }
      event "Suffix:": Value Change {
        n111 = event-data() -> ()  [unwired: 1 in, 6 out]
        n112 = call "Read Channel GUI Array.vi"("error in (no error)"=w280, "SPARC4_GUI in"=w281) -> ("error out"=w284:errorcluster, "Channel GUI Array"=w285:refnum<class "Channel GEI.lvclass">[], "SPARC4_GUI out"=w286:refnum<class "SPARC4_GEI.lvclass">)  [unwired: 7 in]
        n113 = Concatenate Strings("SET SUFFIX ", "Suffix:") -> (w283:string)
        n114 = for {
          tunnel: w285 -> [w304] mode=indexing
          shift-right: [w291] -> w287
          shift-left: w284 -> [w303]
          tunnel: w283 -> [w302]
          tunnel: [w292] -> w282 mode=indexing
          tunnel: "WAIT_DONE" ("Message") -> [w290]
          tunnel: "False" ("Message") -> [w289]
          n115 = call "Send Message.vi"("error in (no error)"=w303, "Message"=w302, "Channel GUI in"=w304) -> ("error out"=w293:errorcluster, "Channel GUI out"=w294:refnum<class "Channel GEI.lvclass">)  [unwired: 7 in]
          n116 = call "Read State Machine.lvclass.vi"("error in (no error)"=w293, "Channel GUI in"=w294) -> ("error out"=w300:errorcluster, "State Machine.lvclass"=w295:refnum<class "State Machine.lvclass">, "Channel GUI out"=w301:refnum<class "Channel GEI.lvclass">)  [unwired: 7 in]
          n117 = call-dynamic "Write State.vi"("error in (no error)"=w300, "State"=w290, "State Machine in"=w295) -> ("error out"=w299:errorcluster, "State Machine out"=w296:refnum<class "State Machine.lvclass">)  [unwired: 7 in]
          n118 = call "Write Next State.vi"("error in (no error)"=w299, "Next State"=w289, "State Machine in"=w296) -> ("error out"=w298:errorcluster, "State Machine out"=w297:refnum<class "State Machine.lvclass">)  [unwired: 7 in]
          n119 = call "Write State Machine.lvclass.vi"("error in (no error)"=w298, "State Machine.lvclass"=w297, "Channel GUI in"=w301) -> ("error out"=w291:errorcluster, "Channel GUI out"=w292:refnum<class "Channel GEI.lvclass">)  [unwired: 7 in]
        }
        n120 = call "Write Channel GUI Array.vi"("error in (no error)"=w287, "Channel GUI Array"=w282, "SPARC4_GUI in"=w286) -> ("error out"=w278:errorcluster, "SPARC4_GUI out"=w279:refnum<class "SPARC4_GEI.lvclass">)  [unwired: 7 in]
      }
      event "Comment:": Value Change {
        n121 = event-data() -> ()  [unwired: 1 in, 1 out]
        n122 = call "Read Channel GUI Array.vi"("error in (no error)"=w310, "SPARC4_GUI in"=w311) -> ("error out"=w314:errorcluster, "Channel GUI Array"=w315:refnum<class "Channel GEI.lvclass">[], "SPARC4_GUI out"=w316:refnum<class "SPARC4_GEI.lvclass">)  [unwired: 7 in]
        n123 = Concatenate Strings("SET COMMENT ", "Comment:") -> (w313:string)
        n124 = for {
          tunnel: w315 -> [w334] mode=indexing
          shift-right: [w322] -> w317
          shift-left: w314 -> [w333]
          tunnel: w313 -> [w332]
          tunnel: [w321] -> w312 mode=indexing
          tunnel: "WAIT_DONE" ("Message") -> [w320]
          tunnel: "False" ("Message") -> [w319]
          n125 = call "Send Message.vi"("error in (no error)"=w333, "Message"=w332, "Channel GUI in"=w334) -> ("error out"=w323:errorcluster, "Channel GUI out"=w324:refnum<class "Channel GEI.lvclass">)  [unwired: 7 in]
          n126 = call "Read State Machine.lvclass.vi"("error in (no error)"=w323, "Channel GUI in"=w324) -> ("error out"=w330:errorcluster, "State Machine.lvclass"=w325:refnum<class "State Machine.lvclass">, "Channel GUI out"=w331:refnum<class "Channel GEI.lvclass">)  [unwired: 7 in]
          n127 = call-dynamic "Write State.vi"("error in (no error)"=w330, "State"=w320, "State Machine in"=w325) -> ("error out"=w329:errorcluster, "State Machine out"=w326:refnum<class "State Machine.lvclass">)  [unwired: 7 in]
          n128 = call "Write Next State.vi"("error in (no error)"=w329, "Next State"=w319, "State Machine in"=w326) -> ("error out"=w328:errorcluster, "State Machine out"=w327:refnum<class "State Machine.lvclass">)  [unwired: 7 in]
          n129 = call "Write State Machine.lvclass.vi"("error in (no error)"=w328, "State Machine.lvclass"=w327, "Channel GUI in"=w331) -> ("error out"=w322:errorcluster, "Channel GUI out"=w321:refnum<class "Channel GEI.lvclass">)  [unwired: 7 in]
        }
        n130 = call "Write Channel GUI Array.vi"("error in (no error)"=w317, "Channel GUI Array"=w312, "SPARC4_GUI in"=w316) -> ("error out"=w308:errorcluster, "SPARC4_GUI out"=w309:refnum<class "SPARC4_GEI.lvclass">)  [unwired: 7 in]
      }
      event "ZERO": Value Change {
        w337 = FALSE
        n131 = event-data() -> ()  [unwired: 1 in, 3 out]
        n132 = Select(t="ZERO", s="ZERO", f="") -> (s? t:f=w338:string)
        n133 = call "Read Channel GUI Array.vi"("error in (no error)"=w349, "SPARC4_GUI in"=w350) -> ("error out"=w352:errorcluster, "Channel GUI Array"=w353:refnum<class "Channel GEI.lvclass">[], "SPARC4_GUI out"=w340:refnum<class "SPARC4_GEI.lvclass">)  [unwired: 7 in]
        n134 = local write "Suffix:"(w338) -> ()
        n135 = Concatenate Strings("SET OBSTYPE ", w338) -> (w342:string)
        n136 = Concatenate Strings("SET SUFFIX ", w338) -> (w341:string)
        n137 = Build Array(w342, w341) -> (w339:string[])
        n138 = for {
          tunnel: w353 -> [w362] mode=indexing
          shift-right: [w360] -> w354
          shift-left: w352 -> [w359]
          tunnel: [w361] -> w351 mode=indexing
          tunnel: w339 -> [w358]
          tunnel: "WAIT_DONE" ("Message") -> [w357]
          tunnel: "False" ("Message") -> [w356]
          n139 = for {
            shift-right: [w366] -> w361
            shift-left: w362 -> [w378]
            shift-right: [w365] -> w360
            shift-left: w359 -> [w377]
            tunnel: w358 -> [w376] mode=indexing
            tunnel: w357 -> [w364]
            tunnel: w356 -> [w363]
            n140 = call "Send Message.vi"("error in (no error)"=w377, "Message"=w376, "Channel GUI in"=w378) -> ("error out"=w367:errorcluster, "Channel GUI out"=w368:refnum<class "Channel GEI.lvclass">)  [unwired: 7 in]
            n141 = call "Read State Machine.lvclass.vi"("error in (no error)"=w367, "Channel GUI in"=w368) -> ("error out"=w374:errorcluster, "State Machine.lvclass"=w369:refnum<class "State Machine.lvclass">, "Channel GUI out"=w375:refnum<class "Channel GEI.lvclass">)  [unwired: 7 in]
            n142 = call-dynamic "Write State.vi"("error in (no error)"=w374, "State"=w364, "State Machine in"=w369) -> ("error out"=w373:errorcluster, "State Machine out"=w370:refnum<class "State Machine.lvclass">)  [unwired: 7 in]
            n143 = call "Write Next State.vi"("error in (no error)"=w373, "Next State"=w363, "State Machine in"=w370) -> ("error out"=w372:errorcluster, "State Machine out"=w371:refnum<class "State Machine.lvclass">)  [unwired: 7 in]
            n144 = call "Write State Machine.lvclass.vi"("error in (no error)"=w372, "State Machine.lvclass"=w371, "Channel GUI in"=w375) -> ("error out"=w365:errorcluster, "Channel GUI out"=w366:refnum<class "Channel GEI.lvclass">)  [unwired: 7 in]
          }
        }
        n145 = call "Write Channel GUI Array.vi"("error in (no error)"=w354, "Channel GUI Array"=w351, "SPARC4_GUI in"=w340) -> ("error out"=w347:errorcluster, "SPARC4_GUI out"=w348:refnum<class "SPARC4_GEI.lvclass">)  [unwired: 7 in]
        n146 = local write "FLAT"(w337) -> ()
        n147 = local write "TEST"(w337) -> ()
        n148 = local write "FOCUS"(w337) -> ()
        n149 = local write "OBJECT"(w337) -> ()
        n150 = local write "DARK"(w337) -> ()
      }
      event "FLAT": Value Change {
        w382 = FALSE
        n151 = event-data() -> ()  [unwired: 1 in, 3 out]
        n152 = Select(t="FLAT", s="FLAT", f="") -> (s? t:f=w383:string)
        n153 = call "Read Channel GUI Array.vi"("error in (no error)"=w393, "SPARC4_GUI in"=w394) -> ("error out"=w396:errorcluster, "Channel GUI Array"=w397:refnum<class "Channel GEI.lvclass">[], "SPARC4_GUI out"=w385:refnum<class "SPARC4_GEI.lvclass">)  [unwired: 7 in]
        n154 = local write "Suffix:"(w383) -> ()
        n155 = Concatenate Strings("SET OBSTYPE ", w383) -> (w387:string)
        n156 = Concatenate Strings("SET SUFFIX ", w383) -> (w386:string)
        n157 = Build Array(w387, w386) -> (w384:string[])
        n158 = for {
          tunnel: w397 -> [w406] mode=indexing
          shift-right: [w404] -> w398
          shift-left: w396 -> [w403]
          tunnel: [w405] -> w395 mode=indexing
          tunnel: w384 -> [w402]
          tunnel: "WAIT_DONE" ("Message") -> [w401]
          tunnel: "False" ("Message") -> [w400]
          n159 = for {
            shift-right: [w410] -> w405
            shift-left: w406 -> [w422]
            shift-right: [w409] -> w404
            shift-left: w403 -> [w421]
            tunnel: w402 -> [w420] mode=indexing
            tunnel: w401 -> [w408]
            tunnel: w400 -> [w407]
            n160 = call "Send Message.vi"("error in (no error)"=w421, "Message"=w420, "Channel GUI in"=w422) -> ("error out"=w411:errorcluster, "Channel GUI out"=w412:refnum<class "Channel GEI.lvclass">)  [unwired: 7 in]
            n161 = call "Read State Machine.lvclass.vi"("error in (no error)"=w411, "Channel GUI in"=w412) -> ("error out"=w418:errorcluster, "State Machine.lvclass"=w413:refnum<class "State Machine.lvclass">, "Channel GUI out"=w419:refnum<class "Channel GEI.lvclass">)  [unwired: 7 in]
            n162 = call-dynamic "Write State.vi"("error in (no error)"=w418, "State"=w408, "State Machine in"=w413) -> ("error out"=w417:errorcluster, "State Machine out"=w414:refnum<class "State Machine.lvclass">)  [unwired: 7 in]
            n163 = call "Write Next State.vi"("error in (no error)"=w417, "Next State"=w407, "State Machine in"=w414) -> ("error out"=w416:errorcluster, "State Machine out"=w415:refnum<class "State Machine.lvclass">)  [unwired: 7 in]
            n164 = call "Write State Machine.lvclass.vi"("error in (no error)"=w416, "State Machine.lvclass"=w415, "Channel GUI in"=w419) -> ("error out"=w409:errorcluster, "Channel GUI out"=w410:refnum<class "Channel GEI.lvclass">)  [unwired: 7 in]
          }
        }
        n165 = call "Write Channel GUI Array.vi"("error in (no error)"=w398, "Channel GUI Array"=w395, "SPARC4_GUI in"=w385) -> ("error out"=w391:errorcluster, "SPARC4_GUI out"=w392:refnum<class "SPARC4_GEI.lvclass">)  [unwired: 7 in]
        n166 = local write "ZERO"(w382) -> ()
        n167 = local write "TEST"(w382) -> ()
        n168 = local write "FOCUS"(w382) -> ()
        n169 = local write "OBJECT"(w382) -> ()
        n170 = local write "DARK"(w382) -> ()
      }
      event "DARK": Value Change {
        w426 = FALSE
        n171 = event-data() -> ()  [unwired: 1 in, 3 out]
        n172 = Select(t="DARK", s="DARK", f="") -> (s? t:f=w427:string)
        n173 = call "Read Channel GUI Array.vi"("error in (no error)"=w437, "SPARC4_GUI in"=w438) -> ("error out"=w440:errorcluster, "Channel GUI Array"=w441:refnum<class "Channel GEI.lvclass">[], "SPARC4_GUI out"=w429:refnum<class "SPARC4_GEI.lvclass">)  [unwired: 7 in]
        n174 = local write "Suffix:"(w427) -> ()
        n175 = Concatenate Strings("SET OBSTYPE ", w427) -> (w431:string)
        n176 = Concatenate Strings("SET SUFFIX ", w427) -> (w430:string)
        n177 = Build Array(w431, w430) -> (w428:string[])
        n178 = for {
          tunnel: w441 -> [w450] mode=indexing
          shift-right: [w448] -> w442
          shift-left: w440 -> [w447]
          tunnel: [w449] -> w439 mode=indexing
          tunnel: w428 -> [w446]
          tunnel: "WAIT_DONE" ("Message") -> [w445]
          tunnel: "False" ("Message") -> [w444]
          n179 = for {
            shift-right: [w454] -> w449
            shift-left: w450 -> [w466]
            shift-right: [w453] -> w448
            shift-left: w447 -> [w465]
            tunnel: w446 -> [w464] mode=indexing
            tunnel: w445 -> [w452]
            tunnel: w444 -> [w451]
            n180 = call "Send Message.vi"("error in (no error)"=w465, "Message"=w464, "Channel GUI in"=w466) -> ("error out"=w455:errorcluster, "Channel GUI out"=w456:refnum<class "Channel GEI.lvclass">)  [unwired: 7 in]
            n181 = call "Read State Machine.lvclass.vi"("error in (no error)"=w455, "Channel GUI in"=w456) -> ("error out"=w462:errorcluster, "State Machine.lvclass"=w457:refnum<class "State Machine.lvclass">, "Channel GUI out"=w463:refnum<class "Channel GEI.lvclass">)  [unwired: 7 in]
            n182 = call-dynamic "Write State.vi"("error in (no error)"=w462, "State"=w452, "State Machine in"=w457) -> ("error out"=w461:errorcluster, "State Machine out"=w458:refnum<class "State Machine.lvclass">)  [unwired: 7 in]
            n183 = call "Write Next State.vi"("error in (no error)"=w461, "Next State"=w451, "State Machine in"=w458) -> ("error out"=w460:errorcluster, "State Machine out"=w459:refnum<class "State Machine.lvclass">)  [unwired: 7 in]
            n184 = call "Write State Machine.lvclass.vi"("error in (no error)"=w460, "State Machine.lvclass"=w459, "Channel GUI in"=w463) -> ("error out"=w453:errorcluster, "Channel GUI out"=w454:refnum<class "Channel GEI.lvclass">)  [unwired: 7 in]
          }
        }
        n185 = call "Write Channel GUI Array.vi"("error in (no error)"=w442, "Channel GUI Array"=w439, "SPARC4_GUI in"=w429) -> ("error out"=w435:errorcluster, "SPARC4_GUI out"=w436:refnum<class "SPARC4_GEI.lvclass">)  [unwired: 7 in]
        n186 = local write "ZERO"(w426) -> ()
        n187 = local write "TEST"(w426) -> ()
        n188 = local write "FOCUS"(w426) -> ()
        n189 = local write "OBJECT"(w426) -> ()
        n190 = local write "FLAT"(w426) -> ()
      }
      event "FOCUS": Value Change {
        w470 = FALSE
        n191 = event-data() -> ()  [unwired: 1 in, 3 out]
        n192 = Select(t="FOCUS", s="FOCUS", f="") -> (s? t:f=w471:string)
        n193 = call "Read Channel GUI Array.vi"("error in (no error)"=w481, "SPARC4_GUI in"=w482) -> ("error out"=w484:errorcluster, "Channel GUI Array"=w485:refnum<class "Channel GEI.lvclass">[], "SPARC4_GUI out"=w473:refnum<class "SPARC4_GEI.lvclass">)  [unwired: 7 in]
        n194 = local write "Suffix:"(w471) -> ()
        n195 = Concatenate Strings("SET OBSTYPE ", w471) -> (w475:string)
        n196 = Concatenate Strings("SET SUFFIX ", w471) -> (w474:string)
        n197 = Build Array(w475, w474) -> (w472:string[])
        n198 = for {
          tunnel: w485 -> [w494] mode=indexing
          shift-right: [w492] -> w486
          shift-left: w484 -> [w491]
          tunnel: [w493] -> w483 mode=indexing
          tunnel: w472 -> [w490]
          tunnel: "WAIT_DONE" ("Message") -> [w489]
          tunnel: "False" ("Message") -> [w488]
          n199 = for {
            shift-right: [w498] -> w493
            shift-left: w494 -> [w510]
            shift-right: [w497] -> w492
            shift-left: w491 -> [w509]
            tunnel: w490 -> [w508] mode=indexing
            tunnel: w489 -> [w496]
            tunnel: w488 -> [w495]
            n200 = call "Send Message.vi"("error in (no error)"=w509, "Message"=w508, "Channel GUI in"=w510) -> ("error out"=w499:errorcluster, "Channel GUI out"=w500:refnum<class "Channel GEI.lvclass">)  [unwired: 7 in]
            n201 = call "Read State Machine.lvclass.vi"("error in (no error)"=w499, "Channel GUI in"=w500) -> ("error out"=w506:errorcluster, "State Machine.lvclass"=w501:refnum<class "State Machine.lvclass">, "Channel GUI out"=w507:refnum<class "Channel GEI.lvclass">)  [unwired: 7 in]
            n202 = call-dynamic "Write State.vi"("error in (no error)"=w506, "State"=w496, "State Machine in"=w501) -> ("error out"=w505:errorcluster, "State Machine out"=w502:refnum<class "State Machine.lvclass">)  [unwired: 7 in]
            n203 = call "Write Next State.vi"("error in (no error)"=w505, "Next State"=w495, "State Machine in"=w502) -> ("error out"=w504:errorcluster, "State Machine out"=w503:refnum<class "State Machine.lvclass">)  [unwired: 7 in]
            n204 = call "Write State Machine.lvclass.vi"("error in (no error)"=w504, "State Machine.lvclass"=w503, "Channel GUI in"=w507) -> ("error out"=w497:errorcluster, "Channel GUI out"=w498:refnum<class "Channel GEI.lvclass">)  [unwired: 7 in]
          }
        }
        n205 = call "Write Channel GUI Array.vi"("error in (no error)"=w486, "Channel GUI Array"=w483, "SPARC4_GUI in"=w473) -> ("error out"=w479:errorcluster, "SPARC4_GUI out"=w480:refnum<class "SPARC4_GEI.lvclass">)  [unwired: 7 in]
        n206 = local write "ZERO"(w470) -> ()
        n207 = local write "TEST"(w470) -> ()
        n208 = local write "OBJECT"(w470) -> ()
        n209 = local write "FLAT"(w470) -> ()
        n210 = local write "FLAT"(w470) -> ()
      }
      event "TEST": Value Change {
        w514 = FALSE
        n211 = event-data() -> ()  [unwired: 1 in, 3 out]
        n212 = Select(t="TEST", s="TEST", f="") -> (s? t:f=w515:string)
        n213 = call "Read Channel GUI Array.vi"("error in (no error)"=w525, "SPARC4_GUI in"=w526) -> ("error out"=w528:errorcluster, "Channel GUI Array"=w529:refnum<class "Channel GEI.lvclass">[], "SPARC4_GUI out"=w517:refnum<class "SPARC4_GEI.lvclass">)  [unwired: 7 in]
        n214 = local write "Suffix:"(w515) -> ()
        n215 = Concatenate Strings("SET OBSTYPE ", w515) -> (w519:string)
        n216 = Concatenate Strings("SET SUFFIX ", w515) -> (w518:string)
        n217 = Build Array(w519, w518) -> (w516:string[])
        n218 = for {
          tunnel: w529 -> [w538] mode=indexing
          shift-right: [w536] -> w530
          shift-left: w528 -> [w535]
          tunnel: [w537] -> w527 mode=indexing
          tunnel: w516 -> [w534]
          tunnel: "WAIT_DONE" ("Message") -> [w533]
          tunnel: "False" ("Message") -> [w532]
          n219 = for {
            shift-right: [w542] -> w537
            shift-left: w538 -> [w554]
            shift-right: [w541] -> w536
            shift-left: w535 -> [w553]
            tunnel: w534 -> [w552] mode=indexing
            tunnel: w533 -> [w540]
            tunnel: w532 -> [w539]
            n220 = call "Send Message.vi"("error in (no error)"=w553, "Message"=w552, "Channel GUI in"=w554) -> ("error out"=w543:errorcluster, "Channel GUI out"=w544:refnum<class "Channel GEI.lvclass">)  [unwired: 7 in]
            n221 = call "Read State Machine.lvclass.vi"("error in (no error)"=w543, "Channel GUI in"=w544) -> ("error out"=w550:errorcluster, "State Machine.lvclass"=w545:refnum<class "State Machine.lvclass">, "Channel GUI out"=w551:refnum<class "Channel GEI.lvclass">)  [unwired: 7 in]
            n222 = call-dynamic "Write State.vi"("error in (no error)"=w550, "State"=w540, "State Machine in"=w545) -> ("error out"=w549:errorcluster, "State Machine out"=w546:refnum<class "State Machine.lvclass">)  [unwired: 7 in]
            n223 = call "Write Next State.vi"("error in (no error)"=w549, "Next State"=w539, "State Machine in"=w546) -> ("error out"=w548:errorcluster, "State Machine out"=w547:refnum<class "State Machine.lvclass">)  [unwired: 7 in]
            n224 = call "Write State Machine.lvclass.vi"("error in (no error)"=w548, "State Machine.lvclass"=w547, "Channel GUI in"=w551) -> ("error out"=w541:errorcluster, "Channel GUI out"=w542:refnum<class "Channel GEI.lvclass">)  [unwired: 7 in]
          }
        }
        n225 = call "Write Channel GUI Array.vi"("error in (no error)"=w530, "Channel GUI Array"=w527, "SPARC4_GUI in"=w517) -> ("error out"=w523:errorcluster, "SPARC4_GUI out"=w524:refnum<class "SPARC4_GEI.lvclass">)  [unwired: 7 in]
        n226 = local write "ZERO"(w514) -> ()
        n227 = local write "DARK"(w514) -> ()
        n228 = local write "OBJECT"(w514) -> ()
        n229 = local write "FLAT"(w514) -> ()
        n230 = local write "FLAT"(w514) -> ()
      }
      event "OBJECT": Value Change {
        w559 = FALSE
        w555 = ""
        n231 = event-data() -> ()  [unwired: 1 in, 3 out]
        n232 = call "Read Channel GUI Array.vi"("error in (no error)"=w567, "SPARC4_GUI in"=w568) -> ("error out"=w570:errorcluster, "Channel GUI Array"=w571:refnum<class "Channel GEI.lvclass">[], "SPARC4_GUI out"=w561:refnum<class "SPARC4_GEI.lvclass">)  [unwired: 7 in]
        n233 = local write "Suffix:"(w555) -> ()
        n234 = Concatenate Strings("SET OBSTYPE ", "OBJECT") -> (w563:string)
        n235 = Concatenate Strings("SET SUFFIX ", w555) -> (w562:string)
        n236 = Build Array(w563, w562) -> (w560:string[])
        n237 = for {
          tunnel: w571 -> [w580] mode=indexing
          shift-right: [w578] -> w572
          shift-left: w570 -> [w577]
          tunnel: [w579] -> w569 mode=indexing
          tunnel: w560 -> [w576]
          tunnel: "WAIT_DONE" ("Message") -> [w575]
          tunnel: "False" ("Message") -> [w574]
          n238 = for {
            shift-right: [w584] -> w579
            shift-left: w580 -> [w596]
            shift-right: [w583] -> w578
            shift-left: w577 -> [w595]
            tunnel: w576 -> [w594] mode=indexing
            tunnel: w575 -> [w582]
            tunnel: w574 -> [w581]
            n239 = call "Send Message.vi"("error in (no error)"=w595, "Message"=w594, "Channel GUI in"=w596) -> ("error out"=w585:errorcluster, "Channel GUI out"=w586:refnum<class "Channel GEI.lvclass">)  [unwired: 7 in]
            n240 = call "Read State Machine.lvclass.vi"("error in (no error)"=w585, "Channel GUI in"=w586) -> ("error out"=w592:errorcluster, "State Machine.lvclass"=w587:refnum<class "State Machine.lvclass">, "Channel GUI out"=w593:refnum<class "Channel GEI.lvclass">)  [unwired: 7 in]
            n241 = call-dynamic "Write State.vi"("error in (no error)"=w592, "State"=w582, "State Machine in"=w587) -> ("error out"=w591:errorcluster, "State Machine out"=w588:refnum<class "State Machine.lvclass">)  [unwired: 7 in]
            n242 = call "Write Next State.vi"("error in (no error)"=w591, "Next State"=w581, "State Machine in"=w588) -> ("error out"=w590:errorcluster, "State Machine out"=w589:refnum<class "State Machine.lvclass">)  [unwired: 7 in]
            n243 = call "Write State Machine.lvclass.vi"("error in (no error)"=w590, "State Machine.lvclass"=w589, "Channel GUI in"=w593) -> ("error out"=w583:errorcluster, "Channel GUI out"=w584:refnum<class "Channel GEI.lvclass">)  [unwired: 7 in]
          }
        }
        n244 = call "Write Channel GUI Array.vi"("error in (no error)"=w572, "Channel GUI Array"=w569, "SPARC4_GUI in"=w561) -> ("error out"=w565:errorcluster, "SPARC4_GUI out"=w566:refnum<class "SPARC4_GEI.lvclass">)  [unwired: 7 in]
        n245 = local write "ZERO"(w559) -> ()
        n246 = local write "TEST"(w559) -> ()
        n247 = local write "FOCUS"(w559) -> ()
        n248 = local write "FLAT"(w559) -> ()
        n249 = local write "DARK"(w559) -> ()
      }
    }
    n250 = Unbundle By Name(w10) -> ("status"=w17:bool)
    n251 = Or(x=w17, y="Stop Application") -> (x .or. y?=w18:bool)
    n252 = call "Erase Message.vi"("error in (no error)"=w10, "SPARC4_GUI in"=w11) -> ("error out"=w13:errorcluster, "SPARC4_GUI out"=w12:refnum<class "SPARC4_GEI.lvclass">)  [unwired: 8 in]
  }
  n253 = Unbundle By Name(w4) -> ("source"=→"Error Message":string)
  n254 = call "End.vi"("SPARC4_GUI in"=w5) -> ("SPARC4_GUI out"=w6:refnum<class "SPARC4_GEI.lvclass">)  [unwired: 9 in, 1 out]
  n255 = flat-sequence {
    tunnel: w6 -> [_]
    frame #0 {
      w597 = u16 0 items=["Clear", "U", "B", "V", "R", "I"] ("Filter")
      w600 = ""
      w599 = FALSE ("Exposing")
      w601 = u16 0 items=["Internal", "External", "N/A", "N/A", "N/A", "N/A", "External Start", "External Exposure (Bulb)", "N/A", "External FVB EM", "Software", "N/A", "External Charge Shifting"] ("Trigger Mode")
      w602 = u16 4 items=["Full Vertical Binning", "Multi-Track", "Random-Track", "Single-Track", "Image"] ("Read Mode")
      w603 = u16 3 items=["Reserved", "Single Scan", "Accumulate", "Kinetic", "Fast Kinetic", "Run till abort", "Reserved", "Reserved", "Reserved", "Time Delayed Integration"] ("Acquisition Mode")
      w608 = u16 0 items=["TTL Low", "TTL High"] ("Shutter TTL")
      w610 = u8 0 items=["  1 MHz", "0.1 MHz"] ("Readout Rate")
      w612 = i16 0 ("Temperature 2")
      w616 = u8 2 items=["Fully Auto", "OPEN", "CLOSED"] ("Shutter Mode")
      w613 = "" ("Command:")
      w618 = u16 1024 ("Final Line")
      w617 = u16 1 ("Initial Cloumn")
      w621 = u8 0 items=["Gain 1", "Gain 2"] ("Pre-amp gain")
      w623 = u16 0 items=["Cooler OFF", "Cooler ON"] ("Cooler ON/OFF")
      w626 = u8 1 items=["Electron Multiplying", "Conventional"] ("EM Mode")
      w614 = "" ("Temperature Status")
      n256 = local write "Camera On/Off"(FALSE ("Initialization")) -> ()
      n257 = local write "Command:"(w613) -> ()
      n258 = local write "Response:"(w613) -> ()
      n259 = local write "Temperature"(20 ("Temperature")) -> ()
      n260 = local write "Temperature Status"(w614) -> ()
      n261 = local write "Exposing"(FALSE ("Exposing")) -> ()
      n262 = local write "Exposições realizadas"(u8 1 ("Exposições realizadas")) -> ()
      n263 = local write "Shutter Mode"(w616) -> ()
      n264 = local write "Exposure Time"(1.0 ("Exposure Time 2")) -> ()
      n265 = local write "Cubes"(u32 1 ("# Ciclos")) -> ()
      n266 = local write "Exp Time"(1.0 ("% Acquired")) -> ()
      n267 = local write "CCD Status"(w614) -> ()
      n268 = local write "Last image"(w613) -> ()
      n269 = property on="Exposições realizadas" class="Slide (strict)"("Scale.Maximum"=1.0 ("Scale.Range:Maximum")) -> ()  [unwired: 2 in, 2 out]
      n270 = property on="Readout Rate" class="Ring (strict)"("Strings []"=string[] ["1 MHz", "0.1 MHz"]) -> ()  [unwired: 2 in, 2 out]
      n271 = local write "Serial Number"(w612) -> ()
      n272 = local write "Temperature"(w612) -> ()
      n273 = local write "Exposure Time 2"(1.0 ("Exposure Time")) -> ()
      n274 = local write "EM Gain"(u16 2 ("EM Gain")) -> ()
      n275 = local write "EM Mode"(w626) -> ()
      n276 = local write "Cooler ON/OFF"(w623) -> ()
      n277 = local write "Readout Rate"(w610) -> ()
      n278 = local write "Pre-amp gain"(w621) -> ()
      n279 = local write "Sub Image"(T1."1024 x 1024" ("Sub Image")) -> ()
      n280 = local write "Initial Line"(u16 1 ("Initial Line")) -> ()
      n281 = local write "Final Line"(w618) -> ()
      n282 = local write "Final Column"(w618) -> ()
      n283 = local write "Initial Cloumn"(w617) -> ()
      n284 = local write "Binning"(w617) -> ()
      n285 = local write "Temperature 2"(i16 20 ("Set temperature")) -> ()
      n286 = local write "Frames"(u16 1 ("Cube Size  2")) -> ()
      n287 = local write "Frames 2"(u16 1 ("Kinetic Series Length")) -> ()
      n288 = local write "Suffix:"(w600) -> ()
      n289 = local write "Comment:"(w600) -> ()
      n290 = local write "Frame Tansfer"(TRUE ("Frame Tansfer")) -> ()
      n291 = local write "Shutter TTL"(w608) -> ()
      n292 = local write "Shutter Time"(u16 50 ("Shutter Time")) -> ()
      n293 = local write "Vertical Shift Speed"(u16 3 ("Vertical Shift Speed")) -> ()
      n294 = local write "AD Channel"(u16 0 ("AD Channel")) -> ()
      n295 = local write "Vertical Clock Voltagem"(u16 0 ("Vertical Clock Voltagem")) -> ()
      n296 = local write "Acquisition Mode"(w603) -> ()
      n297 = local write "Read Mode"(w602) -> ()
      n298 = local write "Trigger Mode"(w601) -> ()
      n299 = local write "Filter"(w597) -> ()
      n300 = local write "ZERO"(w599) -> ()
      n301 = local write "DARK"(w599) -> ()
      n302 = local write "FLAT"(w599) -> ()
      n303 = local write "FOCUS"(w599) -> ()
      n304 = local write "DARK"(w599) -> ()
      n305 = local write "OBJECT"(w599) -> ()
    }
  }
